vi "Read Selected Channels.vi"(0 "VISA in":refnum<visa-resource-name>, 7 "C##,##DO###":string, 11 "error in":errorcluster) -> (3 "Final Output":string, 4 "VISA out":refnum<visa-resource-name>, 6 "Channel Array":dbl[][](array[numeric]), 8 "Selected Buffer":dbl[](array[numeric]), 10 "First Value":dbl, 14 "Channel Polarity (T: Negative, F: Positive)":bool[](array[boolean]), 15 "error out":errorcluster)   [LabVIEW 2018]
uses:
  <vilib>/Analysis/Matrix/Datatypes/RealMatrix.ctl
  archive/CAEN_SY527 v3/CAEN_SY527/CAEN globals.vi
  <vilib>/Analysis/Matrix/Numeric/Conversions/Matrix To Array - RM.vi
  <vilib>/regexp/Match Regular Expression.xnode
  <vilib>/Analysis/Matrix/NI_Matrix.lvlib
panel:
  out "Buffer Char":string
  out "offset past match":i32
  out "after match":string
  out "whole match":string
  out "before match":string
  out "read buffer":string
  out "Channel":i32
  out "Card":i32
  out "Range":i32
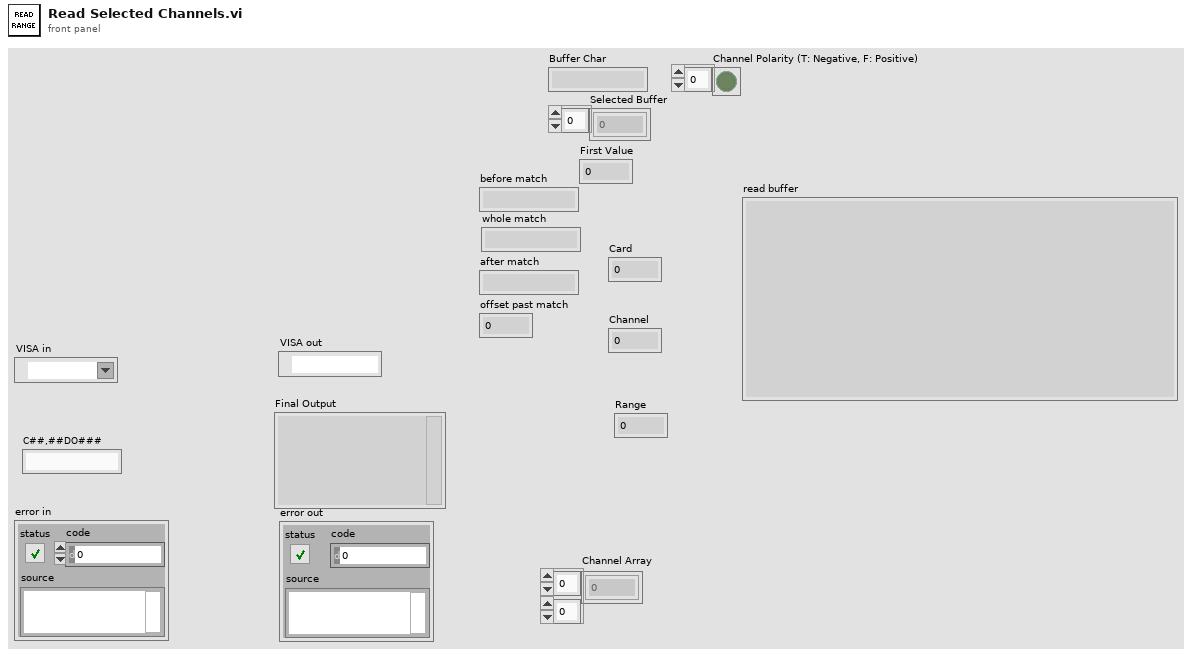
[diagram p1: front panel]
types:
  T1 = typedef "NI_Matrix.lvlib/RealMatrix.ctl" = dbl[][]
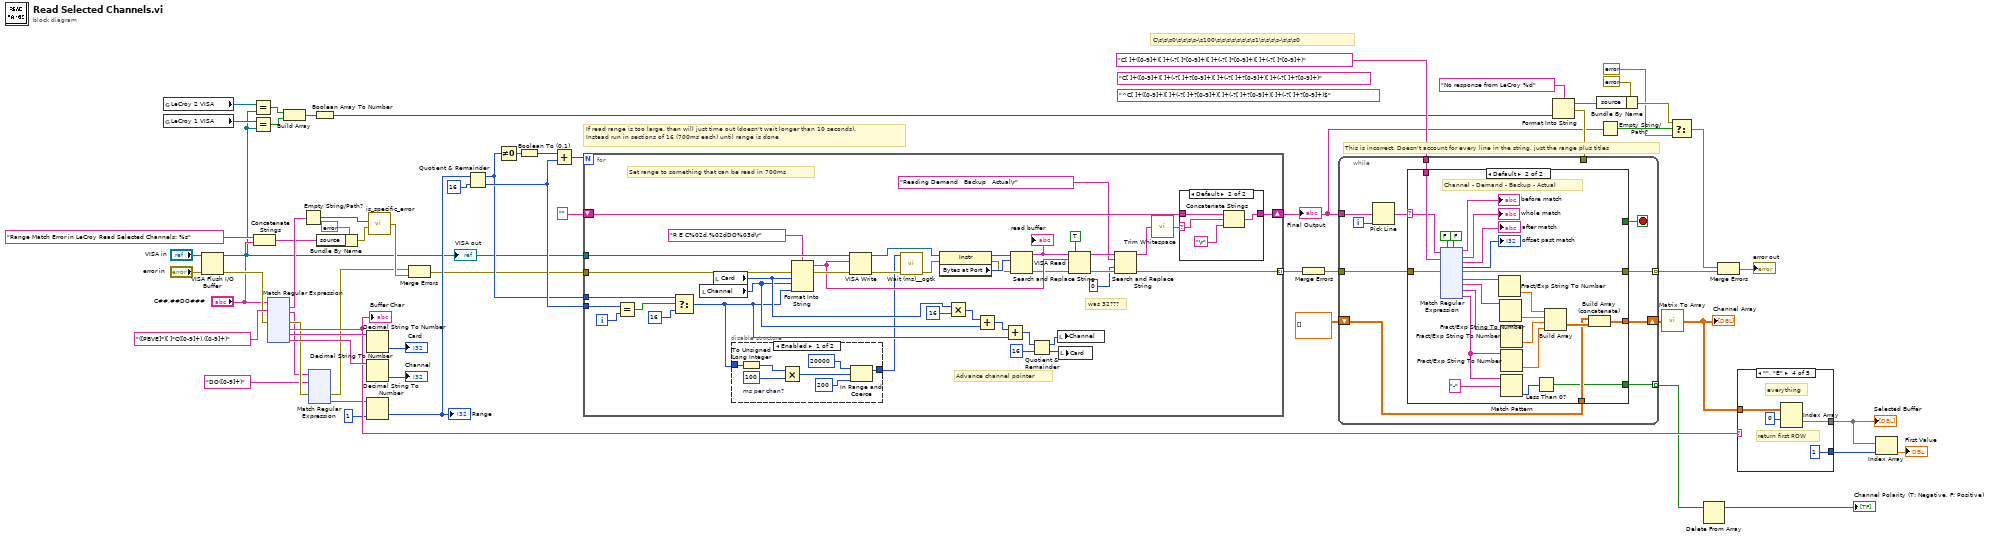
[diagram p0: block diagram]
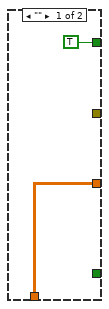
[diagram p2: hidden frame]
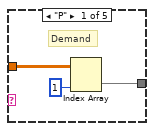
[diagram p3: hidden frame]
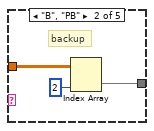
[diagram p4: hidden frame]
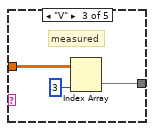
[diagram p5: hidden frame]
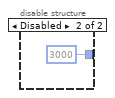
[diagram p8: hidden frame]
diagram:
  (unwired) "C[ ]+([0-9]+)[ ]+(-?[ ]+?[0-9]+)[ ]+(-?[ ]+?[0-9]+)[ ]+(-?[ ]+?[0-9]+)"
  (unwired) "^C[ ]+([0-9]+)[ ]+(-?[ ]+?[0-9]+)[ ]+(-?[ ]+?[0-9]+)[ ]+(-?[ ]+?[0-9]+)$"
  # "This is incorrect. Doesn't account for every line in the string, just the range plus titles"
  # "C\\s\\s\\s0\\s\\s\\s\\s-\\s100\\s\\s\\s\\s\\s\\s\\s\\s1\\s\\s\\s\\s-\\s\\s\\s0"
  # "If read range is too large, then will just time out (doesn't wait longer than 10 seconds).\nInstead run in sections of 16 (700ms each) until range is done"
  n1 = global read "CAEN globals.vi" "LeCroy 2 VISA"() -> (w15:refnum<visa-resource-name>)
  n2 = global read "CAEN globals.vi" "LeCroy 1 VISA"() -> (w14:refnum<visa-resource-name>)
  n3 = VISA Flush I/O Buffer(VISA resource name="VISA in", error in (no error)="error in") -> (VISA resource name out=w13:refnum<visa-resource-name>, error out=w44:errorcluster)  [unwired: 1 in]
  "VISA out" <- w13
  n4 = Equal?(x=w15, y=w13) -> (x = y?=w12:bool)
  n5 = Equal?(x=w14, y=w13) -> (x = y?=w11:bool)
  n6 = Concatenate Strings("Range Match Error in LeCroy Read Selected Channels: %s" ("source"), "C##,##DO###") -> (w26:string)
  n7 = xnode "Match Regular Expression"("input string"="C##,##DO###", "regular expression"="([PBVE]*)[ ]*C([0-9]+),([0-9]+)" ("format string"), "error in"=w44) -> ("whole match"=w29:string, "after match"=w32:string, "error out"=w34:errorcluster, "submatch 1"=w40:string, "submatch 2"=w46:string, "submatch 3"=w45:string)  [unwired: 3 in, 2 out]
  "Buffer Char" <- w40
  n8 = Build Array(w12, w11) -> (w10:bool[])
  n9 = Empty String/Path?(string/path=w29) -> (empty?=w28:bool)
  n10 = xnode "Match Regular Expression"("input string"=w32, "regular expression"="DO([0-9]+)" ("format string"), "error in"=w34) -> ("error out"=w21:errorcluster, "submatch 1"=w31:string)  [unwired: 3 in, 4 out]
  n11 = Boolean Array To Number(Boolean array=w10) -> (number=w9:u32)
  n12 = Bundle By Name(cluster=errorcluster {"status"=TRUE, "code"=0, "source"=""} ("error in (no error)"), "source"=w26) -> (w23:errorcluster)
  n13 = Decimal String To Number(string=w45) -> (number=→"Channel":i32)  [unwired: 2 in, 1 out]
  n14 = Decimal String To Number(string=w46) -> (number=→"Card":i32)  [unwired: 2 in, 1 out]
  n15 = Decimal String To Number(string=w31, default (0L)=1 ("default (0 I32)")) -> (number=w41:i32)  [unwired: 1 in, 1 out]
  "Range" <- w41
  n16 = call "is_specific_error.vi"("Boolean"=w28, "error in (no error)"=w23) -> ("error out"=w22:errorcluster)  [unwired: 6 in]
  n17 = Merge Errors(w21, w22) -> (w20:errorcluster)
  n18 = Quotient & Remainder(x=w41, y=16) -> (x-y*floor(x/y)=w49:i32, floor(x/y)=w57:i32)
  n19 = Not Equal To 0?(x=w49) -> (x != 0?=w56:bool)
  n20 = Boolean To (0,1)(Boolean=w56) -> (0, 1=w55:i16)
  n21 = Add(x=w55, y=w57) -> (x+y=w58:i32)
  n22 = for {
    N: w58 -> [_]
    tunnel: w57 -> [w99]
    tunnel: w13 -> [w97]
    tunnel: w20 -> [w96]
    tunnel: [w94] -> w54 mode=indexing
    tunnel: w49 -> [w93]
    shift-right: [w95] -> w5
    shift-left: "" -> [w92]
    i -> [w100]
    # "was 32???"
    # "Advance channel pointer"
    # "Set range to something that can be read in 700ms"
    n23 = Equal?(x=w99, y=w100) -> (x = y?=w98:bool)
    n24 = Select(t=w93, s=w98, f=16) -> (s? t:f=w88:i32)
    n25 = local read "Channel"() -> (w89:i32)
    n26 = local read "Card"() -> (w90:i32)
    n27 = disable-structure shown="Enabled" {
      disable-tunnel: w88 -> [w112 _]
      disable-tunnel: [w108 u32 3000 ("milliseconds to wait")] -> w72
      frame Enabled {
        w107 = u32 100  # ms per chan?
        n28 = To Unsigned Long Integer(number=w112) -> (unsigned 32bit integer=w106:u32)
        n29 = Multiply(x=w106, y=w107) -> (x*y=w109:u32)
        n30 = In Range and Coerce(upper limit=u32 20000, x=w109, lower limit=u32 200 ("upper limit")) -> (coerced(x)=w108:u32)  [unwired: 1 out]
      }
      frame Disabled {
      }
    }
    n31 = Format Into String(format string="R E C%02d,%02dDO%03d\r", error in=w96, w90, w89, w88) -> (resulting string=w79:string, error out=w86:errorcluster)  [unwired: 1 in]
    n32 = VISA Write(VISA resource name=w97, write buffer=w79, error in (no error)=w86) -> (VISA resource name out=w70:refnum<visa-resource-name>, error out=w85:errorcluster)  [unwired: 1 out]
    n33 = call <userlib>:"Wait (ms)__ogtk.vi"("error in (no error)"=w85, "milliseconds to wait"=w72) -> ("error out"=w84:errorcluster)  [unwired: 8 in, 1 out]
    n34 = property class="Instr"(reference=w70, error in=w84) -> (reference out=w81:refnum<visa-resource-name>, error out=w82:errorcluster, "Bytes at Port"=w83:u32)
    n35 = Multiply(x=w90, y=16) -> (x*y=w65:i32)
    n36 = Add(x=w65, y=w89) -> (x+y=w66:i32)
    n37 = Add(x=w66, y=w88) -> (x+y=w67:i32)
    n38 = VISA Read(VISA resource name=w81, byte count=w83, error in (no error)=w82) -> (read buffer=w78:string, error out=w75:errorcluster)  [unwired: 2 out]
    "read buffer" <- w78
    n39 = Quotient & Remainder(x=w67, y=16) -> (x-y*floor(x/y)=w68:i32, floor(x/y)=w69:i32)
    n40 = local write "Channel"(w68) -> ()
    n41 = local write "Card"(w69) -> ()
    n42 = Search and Replace String(replace all?=TRUE ("replace all? (F)"), input string=w78, search string=w79, error in=w75) -> (result string=w77:string, error out=w76:errorcluster)  [unwired: 4 in, 2 out]
    n43 = Search and Replace String(input string=w77, search string="Reading Demand   Backup   Actual\r", offset=0 ("offset (0)"), error in=w76) -> (result string=w91:string, error out=w94:errorcluster)  [unwired: 4 in, 2 out]
    n44 = call <vilib>:"Trim Whitespace.vi"("string"=w91) -> ("trimmed string"=w62:string)  [unwired: 1 in]
    n45 = case shown="Default" w62 {
      selector: w62 -> [_ w102]
      tunnel: [w101 w105] -> w95
      tunnel: w92 -> [w101 w104]
      frame "" {
      }
      frame Default {
        n46 = Concatenate Strings(w104, w102, "\r") -> (w105:string)
      }
    }
  }
  "Final Output" <- w5
  n47 = Merge Errors(w54) -> (w60:errorcluster)
  n48 = Format Into String(format string="No response from LeCroy %d", w9) -> (resulting string=w7:string, error out=w6:errorcluster)  [unwired: 2 in]
  n49 = while {
    tunnel: w5 -> [w122]
    tunnel: w60 -> [w121]
    tunnel: [w120] -> w53 mode=indexing
    shift-right: [w118] -> w37
    shift-left: T1 [] ("Channel Read as Matrix") -> [w119]
    tunnel: "C[ ]+([0-9]+)[ ]+(-?[ ]*[0-9]+)[ ]+(-?[ ]*[0-9]+)[ ]+(-?[ ]*[0-9]+)" -> [w117]
    tunnel: [w116] -> w19 mode=indexing
    tunnel: w6 -> [_]
    i -> [w123]
    stop <- w114 stop-if-true
    n50 = Pick Line(multi-line string=w122, line index=w123) -> (output string=w115:string)  [unwired: 1 in]
    n51 = case shown="Default" w115 {
      selector: w115 -> [_ w126]
      tunnel: w121 -> [_ w139]
      tunnel: [_ w138] -> w120
      tunnel: w119 -> [w125 w137]
      tunnel: [w125 w136] -> w118
      tunnel: w117 -> [_ w131]
      tunnel: [_ w127] -> w116
      tunnel: [TRUE _] -> w114
      frame "" {
      }
      frame Default {
        # "Channel - Demand - Backup - Actual"
        n52 = xnode "Match Regular Expression"("input string"=w126, "regular expression"=w131, "error in"=w139, "ignore case? (F)"=FALSE, "multiline? (F)"=FALSE) -> ("before match"=→"before match":string, "whole match"=→"whole match":string, "after match"=→"after match":string, "offset past match"=→"offset past match":i32, "error out"=w138:errorcluster, "submatch 1"=w147:string, "submatch 2"=w146:string, "submatch 3"=w145:string, "submatch 4"=w128:string)  [unwired: 1 in]
        n53 = Fract/Exp String To Number(string=w147) -> (number=w144:dbl)  [unwired: 3 in, 1 out]
        n54 = Fract/Exp String To Number(string=w146) -> (number=w143:dbl)  [unwired: 3 in, 1 out]
        n55 = Fract/Exp String To Number(string=w145) -> (number=w142:dbl)  [unwired: 3 in, 1 out]
        n56 = Fract/Exp String To Number(string=w128) -> (number=w141:dbl)  [unwired: 3 in, 1 out]
        n57 = Match Pattern(string=w128, regular expression="-") -> (offset past match=w130:i32)  [unwired: 1 in, 3 out]
        n58 = Less Than 0?(x=w130) -> (x < 0?=w127:bool)
        n59 = Build Array ("Build Matrix")(w144, w143, w142, w141) -> (w140:T1)
        n60 = Build Array (concatenate) ("Build Matrix")(w137, w140) -> (w136:T1)
      }
    }
  }
  n61 = Bundle By Name(cluster=errorcluster {"status"=TRUE, "code"=0, "source"=""} ("error out"), "source"=w7) -> (w3:errorcluster)
  n62 = Empty String/Path?(string/path=w5) -> (empty?=w4:bool)
  n63 = call-poly <vilib>:"Matrix To Array.vi"("Real Matrix"=w37) -> ("Real 2D Array"=w36:dbl[][])
  "Channel Array" <- w36
  n64 = Select(t=w3, s=w4, f=errorcluster {"status"=FALSE, "code"=0, "source"=""} ("error out")) -> (s? t:f=w1:errorcluster)
  n65 = Delete From Array(array=w19) -> (array with subset deleted=→"Channel Polarity (T: Negative, F: Positive)":bool[])  [unwired: 2 in, 1 out]
  n66 = Merge Errors(w1, w53) -> (→"error out":errorcluster)
  n67 = case shown="\"\", \"E\"" w40 {
    tunnel: w36 -> [w271 w274 w277 w281 _]
    tunnel: [w269 w272 w275 w280 _] -> w39
    tunnel: [_ _ _ 1 ("index (row)") _] -> w17
    frame "P" {
      # "Demand"
      n68 = Index Array(array=w271, index (col)=1 ("disabled index (col)")) -> (element=w269:dbl[])  [unwired: 1 in]
    }
    frame "B", "PB" {
      # "backup"
      n69 = Index Array(array=w274, index (col)=2 ("disabled index (col)")) -> (element=w272:dbl[])  [unwired: 1 in]
    }
    frame "V" {
      # "measured"
      n70 = Index Array(array=w277, index (col)=3 ("disabled index (col)")) -> (element=w275:dbl[])  [unwired: 1 in]
    }
    frame "", "E" {
      # "return first ROW"
      # "everything"
      n71 = Index Array(array=w281, index (row)=0) -> (element=w280:dbl[])  [unwired: 1 in]
    }
    frame Default {
      # "??? unknown \nbuffer"
    }
  }
  "Selected Buffer" <- w39
  n72 = Index Array(array=w39, index=w17) -> (element=→"First Value":dbl)
